vi "Read Program Path.vi"(8 "error in":errorcluster, 11 "MPLab in":refnum<class "MPLab.lvclass">) -> (0 "error out":errorcluster, 3 "MPLab out":refnum<class "MPLab.lvclass">)   [LabVIEW 2018, in "MPLab.lvlib" / "MPLab.lvclass"]
uses:
  MPLab.lvclass
  MPLab.lvclass/MPLab.ctl
  builds/Flash Utility.lvlibp/Flash Utility.lvclass
  builds/Configuration.lvlibp/Configuration.lvclass
  C:/Users/Ron.Dexter.LUMINARTECH/Desktop/builds/Flash Utility.lvlibp/Flash Utility.lvclass
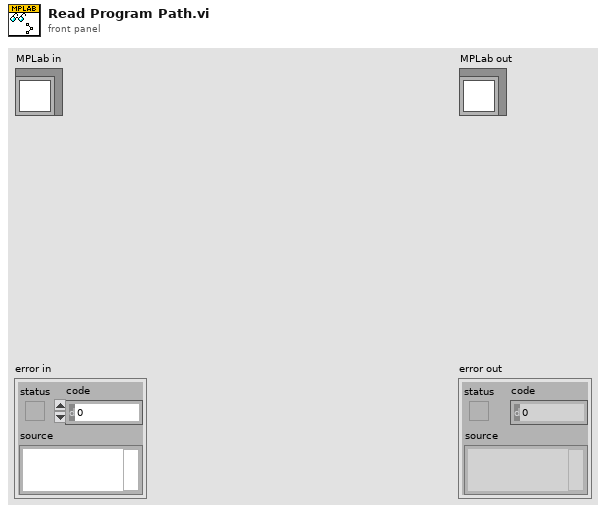
[diagram p1: front panel]
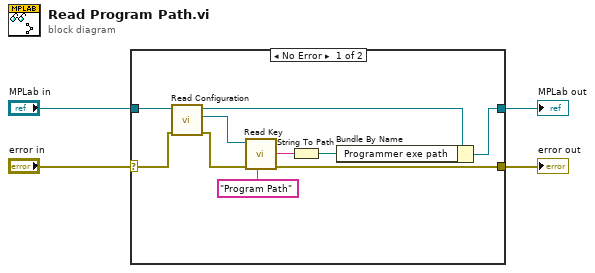
[diagram p0: block diagram]
diagram:
  n1 = case shown="No Error" "error in" {
    selector: "error in" -> [w5 w16]
    tunnel: [w7 w16] -> w3
    tunnel: [w10 w15] -> w1
    tunnel: "MPLab in" -> [w14 w15]
    frame No Error {
      n2 = call "Read Configuration.vi"("error in (no error)"=w5, "Flash Utility in"=w14) -> ("error out"=w6:errorcluster, "Configuration"=w13:refnum<class "Configuration.lvclass">, "Flash Utility out"=w11:refnum<class "MPLab.lvclass">)  [unwired: 7 in]
      n3 = call "Read Key.vi"("Key:"="Program Path", "error in"=w6, "Configuration in"=w13) -> ("error out"=w7:errorcluster, "Value"=w9:string)  [unwired: 6 in, 1 out]
      n4 = String To Path(string=w9) -> (path=w8:path)
      n5 = Bundle By Name(cluster=w11, "Programmer exe path"=w8) -> (w10:refnum<class "MPLab.lvclass">)
    }
    frame Error {
    }
  }
  "error out" <- w3
  "MPLab out" <- w1
